vi "Main UI.vi"() -> ()   [LabVIEW 2021, in "Model.lvlib" / "Model.lvclass"]
uses:
  Model.lvclass
  <vilib>/OPCUA/controls/Subscription Data Change.ctl
  <vilib>/OPCUA/controls/NodeId.ctl
  <vilib>/OPCUA/controls/Data Type.ctl
  <vilib>/OPCUA/controls/OPC UA StatusCode.ctl
  Model.lvclass/Model.ctl
  <userlib>/John_Lib/Control/Panel State.ctl
  4ea6d537-f583-4af7-96b6-6e87ab69176a.vi
  dc795a0a-56a2-4742-a88d-ac9ee3460b1e.vi
  c0b4bdcd-4b65-4d6d-9257-8d5db7939309.vi
  005296f9-3097-4282-8b9c-b94103fb0c3d.vi
  921fea1b-c06a-452a-ac70-ed1835565b05.vi
  3e3e7c9d-885d-4de5-9ea6-85f2850c837d.vi
  cba7e740-a3a4-4717-84ae-86dbe1cc8337.vi
  <userlib>/John_Lib/OPCUA/UA Read Varient.vi
  adfd9d9b-45c5-4f5b-a64f-74c91a2677a3.vi
  <userlib>/John_Lib/AMC_FW/Send Local Message.vi
  <userlib>/John_Lib/AMC_FW/Read Next Message.vi
  <userlib>/John_Lib/AMC_FW/Parse State Queue__JKI.vi
  <userlib>/John_Lib/AMC_FW/Create Single Message.vi
  <userlib>/John_Lib/AMC_FW/Update Message Routing Info.vi
  <userlib>/John_Lib/AMC_FW/Read Termination Message.vi
  <vilib>/Utility/Data Type/Get Type Information.vi
  <userlib>/John_Lib/AMC_FW/String to Array.vi
  <userlib>/John_Lib/String/DBL to String.vi
  <userlib>/John_Lib/AMC_FW/Send Message.vi
  <userlib>/John_Lib/AMC_FW/Globals.vi
  <vilib>/Utility/error.llb/Trim Whitespace.vi
  <userlib>/John_Lib/OPCUA/add NameSpace for single NoteID.vi
  <vilib>/OPCUA/client/internal/Read.vi
  <vilib>/OPCUA/client/internal/Read Variant.vi
  <userlib>/John_Lib/OPCUA/OPCUA.lvclass
  <userlib>/John_Lib/AMC_FW/AMC_FW.lvlib
  <userlib>/John_Lib/TopPath/TopPath.lvlib
panel:
  in  "stop":bool
  out "data change":T1[](array[typedef]) {"data type" items=["Boolean"=1, "SByte"=2, "Byte"=3, "Int16"=4, "UInt16"=5, "Int32"=6, "UInt32"=7, "Int64"=8, "UInt64"=9, "Float"=10, "Double"=11, "String"=12, "DateTime"=13, "ByteString"=15, "Array of Boolean"=101, "Array of SByte"=102, "Array of Byte"=103, "Array of Int16"=104, "Array of UInt16"=105, "Array of Int32"=106, "Array of UInt32"=107, "Array of Int64"=108, "Array of UInt64"=109, "Array of Float"=110, "Array of Double"=111, "Array of String"=112, "Array of DateTime"=113, "Array of ByteString"=115, "Matrix of Boolean"=201, "Matrix of SByte"=202, "Matrix of Byte"=203, "Matrix of Int16"=204, "Matrix of UInt16"=205, "Matrix of Int32"=206, "Matrix of UInt32"=207, "Matrix of Int64"=208, "Matrix of UInt64"=209, "Matrix of Float"=210, "Matrix of Double"=211, "Matrix of String "=212, "Matrix of DateTime"=213, "Matrix of ByteString"=215]; "status code" items=["Good"=0, "Good_SubscriptionTransferred"=2949120, "Good_CompletesAsynchronously"=3014656, "Good_Overload"=3080192, "Good_Clamped"=3145728, "Good_LocalOverride"=9830400, "Good_EntryInserted"=10616832, "Good_EntryReplaced"=10682368, "Good_NoData"=10813440, "Good_MoreData"=10878976, "Good_CommunicationEvent"=10944512, "Good_ShutdownEvent"=11010048, "Good_CallAgain"=11075584, "Good_NonCriticalTimeout"=11141120, "Good_ResultsMayBeIncomplete"=12189696, "Good_DataIgnored"=14221312, "Uncertain"=1073741824, "Uncertain_ReferenceOutOfServer"=1080819712, "Uncertain_NoCommunicationLastUsableValue"=1083113472, "Uncertain_LastUsableValue"=1083179008, "Uncertain_SubstituteValue"=1083244544, "Uncertain_InitialValue"=1083310080, "Uncertain_SensorNotAccurate"=1083375616, "Uncertain_EngineeringUnitsExceeded"=1083441152, "Uncertain_SubNormal"=1083506688, "Uncertain_DataSubNormal"=1084489728, "Uncertain_ReferenceNotDeleted"=1086062592, "Uncertain_NotAllNodesAvailable"=1086324736, "Bad"=2147483648, "Bad_UnexpectedError"=2147549184, "Bad_InternalError"=2147614720, "Bad_OutOfMemory"=2147680256, "Bad_ResourceUnavailable"=2147745792, "Bad_CommunicationError"=2147811328, "Bad_EncodingError"=2147876864, "Bad_DecodingError"=2147942400, "Bad_EncodingLimitsExceeded"=2148007936, "Bad_UnknownResponse"=2148073472, "Bad_Timeout"=2148139008, "Bad_ServiceUnsupported"=2148204544, "Bad_Shutdown"=2148270080, "Bad_ServerNotConnected"=2148335616, "Bad_ServerHalted"=2148401152, "Bad_NothingToDo"=2148466688, "Bad_TooManyOperations"=2148532224, "Bad_DataTypeIdUnknown"=2148597760, "Bad_CertificateInvalid"=2148663296, "Bad_SecurityChecksFailed"=2148728832, "Bad_CertificateTimeInvalid"=2148794368, "Bad_CertificateIssuerTimeInvalid"=2148859904, "Bad_CertificateHostNameInvalid"=2148925440, "Bad_CertificateUriInvalid"=2148990976, "Bad_CertificateUseNotAllowed"=2149056512, "Bad_CertificateIssuerUseNotAllowed"=2149122048, "Bad_CertificateUntrusted"=2149187584, "Bad_CertificateRevocationUnknown"=2149253120, "Bad_CertificateIssuerRevocationUnknown"=2149318656, "Bad_CertificateRevoked"=2149384192, "Bad_CertificateIssuerRevoked"=2149449728, "Bad_UserAccessDenied"=2149515264, "Bad_IdentityTokenInvalid"=2149580800, "Bad_IdentityTokenRejected"=2149646336, "Bad_SecureChannelIdInvalid"=2149711872, "Bad_InvalidTimestamp"=2149777408, "Bad_NonceInvalid"=2149842944, "Bad_SessionIdInvalid"=2149908480, "Bad_SessionClosed"=2149974016, "Bad_SessionNotActivated"=2150039552, "Bad_SubscriptionIdInvalid"=2150105088, "Bad_RequestHeaderInvalid"=2150236160, "Bad_TimestampsToReturnInvalid"=2150301696, "Bad_RequestCancelledByClient"=2150367232, "Bad_NoCommunication"=2150694912, "Bad_WaitingForInitialData"=2150760448, "Bad_NodeIdInvalid"=2150825984, "Bad_NodeIdUnknown"=2150891520, "Bad_AttributeIdInvalid"=2150957056, "Bad_IndexRangeInvalid"=2151022592, "Bad_IndexRangeNoData"=2151088128, "Bad_DataEncodingInvalid"=2151153664, "Bad_DataEncodingUnsupported"=2151219200, "Bad_NotReadable"=2151284736, "Bad_NotWritable"=2151350272, "Bad_OutOfRange"=2151415808, "Bad_NotSupported"=2151481344, "Bad_NotFound"=2151546880, "Bad_ObjectDeleted"=2151612416, "Bad_NotImplemented"=2151677952, "Bad_MonitoringModeInvalid"=2151743488, "Bad_MonitoredItemIdInvalid"=2151809024, "Bad_MonitoredItemFilterInvalid"=2151874560, "Bad_MonitoredItemFilterUnsupported"=2151940096, "Bad_FilterNotAllowed"=2152005632, "Bad_StructureMissing"=2152071168, "Bad_EventFilterInvalid"=2152136704, "Bad_ContentFilterInvalid"=2152202240, "Bad_FilterOperandInvalid"=2152267776, "Bad_ContinuationPointInvalid"=2152333312, "Bad_NoContinuationPoints"=2152398848, "Bad_ReferenceTypeIdInvalid"=2152464384, "Bad_BrowseDirectionInvalid"=2152529920, "Bad_NodeNotInView"=2152595456, "Bad_ServerUriInvalid"=2152660992, "Bad_ServerNameMissing"=2152726528, "Bad_DiscoveryUrlMissing"=2152792064, "Bad_SempahoreFileMissing"=2152857600, "Bad_RequestTypeInvalid"=2152923136, "Bad_SecurityModeRejected"=2152988672, "Bad_SecurityPolicyRejected"=2153054208, "Bad_TooManySessions"=2153119744, "Bad_UserSignatureInvalid"=2153185280, "Bad_ApplicationSignatureInvalid"=2153250816, "Bad_NoValidCertificates"=2153316352, "Bad_RequestCancelledByRequest"=2153381888, "Bad_ParentNodeIdInvalid"=2153447424, "Bad_ReferenceNotAllowed"=2153512960, "Bad_NodeIdRejected"=2153578496, "Bad_NodeIdExists"=2153644032, "Bad_NodeClassInvalid"=2153709568, "Bad_BrowseNameInvalid"=2153775104, "Bad_BrowseNameDuplicated"=2153840640, "Bad_NodeAttributesInvalid"=2153906176, "Bad_TypeDefinitionInvalid"=2153971712, "Bad_SourceNodeIdInvalid"=2154037248, "Bad_TargetNodeIdInvalid"=2154102784, "Bad_DuplicateReferenceNotAllowed"=2154168320, "Bad_InvalidSelfReference"=2154233856, "Bad_ReferenceLocalOnly"=2154299392, "Bad_NoDeleteRights"=2154364928, "Bad_ServerIndexInvalid"=2154430464, "Bad_ViewIdUnknown"=2154496000, "Bad_TooManyMatches"=2154627072, "Bad_QueryTooComplex"=2154692608, "Bad_NoMatch"=2154758144, "Bad_MaxAgeInvalid"=2154823680, "Bad_HistoryOperationInvalid"=2154889216, "Bad_HistoryOperationUnsupported"=2154954752, "Bad_WriteNotSupported"=2155020288, "Bad_TypeMismatch"=2155085824, "Bad_MethodInvalid"=2155151360, "Bad_ArgumentsMissing"=2155216896, "Bad_TooManySubscriptions"=2155282432, "Bad_TooManyPublishRequests"=2155347968, "Bad_NoSubscription"=2155413504, "Bad_SequenceNumberUnknown"=2155479040, "Bad_MessageNotAvailable"=2155544576, "Bad_InsufficientClientProfile"=2155610112, "Bad_TcpServerTooBusy"=2155675648, "Bad_TcpMessageTypeInvalid"=2155741184, "Bad_TcpSecureChannelUnknown"=2155806720, "Bad_TcpMessageTooLarge"=2155872256, "Bad_TcpNotEnoughResources"=2155937792, "Bad_TcpInternalError"=2156003328, "Bad_TcpEndpointUrlInvalid"=2156068864, "Bad_RequestInterrupted"=2156134400, "Bad_RequestTimeout"=2156199936, "Bad_SecureChannelClosed"=2156265472, "Bad_SecureChannelTokenUnknown"=2156331008, "Bad_SequenceNumberInvalid"=2156396544, "Bad_ConfigurationError"=2156462080, "Bad_NotConnected"=2156527616, "Bad_DeviceFailure"=2156593152, "Bad_SensorFailure"=2156658688, "Bad_OutOfService"=2156724224, "Bad_DeadbandFilterInvalid"=2156789760, "Bad_RefreshInProgress"=2157379584, "Bad_ConditionAlreadyDisabled"=2157445120, "Bad_ConditionDisabled"=2157510656, "Bad_EventIdUnknown"=2157576192, "Bad_NoData"=2157641728, "Bad_DataLost"=2157772800, "Bad_DataUnavailable"=2157838336, "Bad_EntryExists"=2157903872, "Bad_NoEntryExists"=2157969408, "Bad_TimestampNotSupported"=2158034944, "Bad_InvalidArgument"=2158690304, "Bad_ConnectionRejected"=2158755840, "Bad_Disconnect"=2158821376, "Bad_ConnectionClosed"=2158886912, "Bad_InvalidState"=2158952448, "Bad_EndOfStream"=2159017984, "Bad_NoDataAvailable"=2159083520, "Bad_WaitingForResponse"=2159149056, "Bad_OperationAbandoned"=2159214592, "Bad_ExpectedStreamToBlock"=2159280128, "Bad_WouldBlock"=2159345664, "Bad_SyntaxError"=2159411200, "Bad_MaxConnectionsReached"=2159476736, "Bad_RequestTooLarge"=2159542272, "Bad_ResponseTooLarge"=2159607808, "Bad_EventNotAcknowledgeable"=2159738880, "Bad_InvalidTimestampArgument"=2159869952, "Bad_ProtocolVersionUnsupported"=2159935488, "Bad_StateNotActive"=2160001024, "Bad_FilterOperatorInvalid"=2160132096, "Bad_FilterOperatorUnsupported"=2160197632, "Bad_FilterOperandCountMismatch"=2160263168, "Bad_FilterElementInvalid"=2160328704, "Bad_FilterLiteralInvalid"=2160394240, "Bad_IdentityChangeNotSupported"=2160459776, "Bad_NotTypeDefinition"=2160590848, "Bad_ViewTimestampInvalid"=2160656384, "Bad_ViewParameterMismatch"=2160721920, "Bad_ViewVersionInvalid"=2160787456, "Bad_ConditionAlreadyEnabled"=2160852992, "Bad_DialogNotActive"=2160918528, "Bad_DialogResponseInvalid"=2160984064, "Bad_ConditionBranchAlreadyAcked"=2161049600, "Bad_ConditionBranchAlreadyConfirmed"=2161115136, "Bad_ConditionAlreadyShelved"=2161180672, "Bad_ConditionNotShelved"=2161246208, "Bad_ShelvingTimeOutOfRange"=2161311744, "Bad_AggregateListMismatch"=2161377280, "Bad_AggregateNotSupported"=2161442816, "Bad_AggregateInvalidInputs"=2161508352, "Bad_BoundNotFound"=2161573888, "Bad_BoundNotSupported"=2161639424, "Bad_AggregateConfigurationRejected"=2161770496, "Bad_TooManyMonitoredItems"=2161836032]}
  out "value":variant
  in  "node ID":string
  in  "error out":errorcluster
  out "Error Out":errorcluster
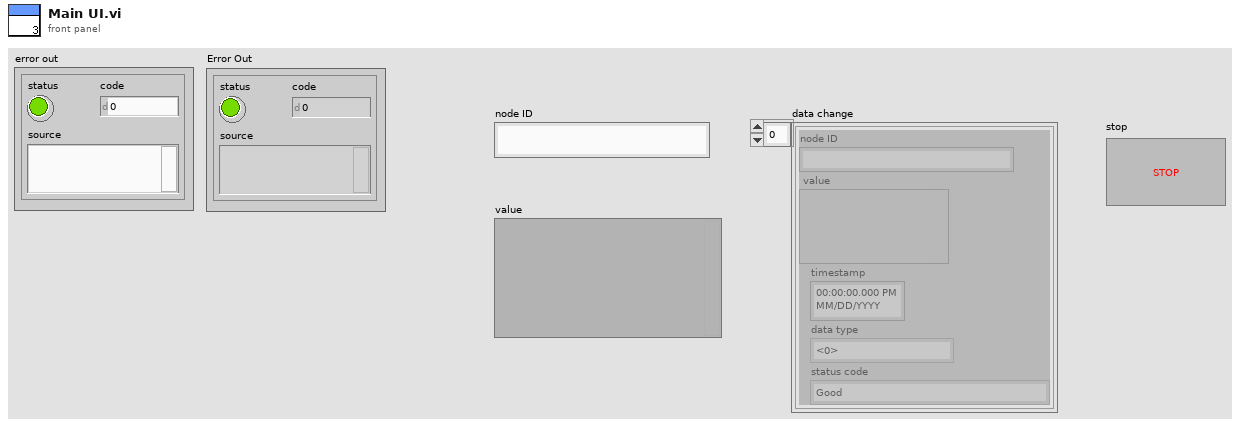
[diagram p1: front panel]
types:
  T1 = typedef "Subscription Data Change.ctl" = cluster{"node ID":T2, " value":variant, "timestamp":timestamp, "data type":T3, "status code":T4}
  T2 = typedef "NodeId.ctl" = string
  T3 = typedef "Data Type.ctl" = u16
  T4 = typedef "OPC UA StatusCode.ctl" = u32
  T5 = typedef "OPCUA.lvlib/OPCUA.lvclass/OPCUA Even.ctl" = cluster{"OPC UA data change":refnum<user-event>, "ReSubscribtion":refnum<user-event>}
  T6 = typedef "Model.lvlib/Model.lvclass/Evens.ctl" = cluster{"NotifyIcon":refnum<user-event>, "Stop":refnum<user-event>}
  T7 = typedef "AMC_FW.lvlib/Queue.ctl" = cluster{"Q":T8, "Name":string}
  T8 = typedef "AMC_FW.lvlib/Message Queue.ctl" = refnum<queue>
  T9 = enum32{"invalid app kind", "Development System", "Run Time System", "Student Edition", "Embedded LabVIEW", "Evaluation", "Custom"}
  T10 = typedef "Panel State.ctl" = string
  T11 = typedef "Model.lvlib/Model.lvclass/DVR.ctl" = cluster{"JKI_Network_Streams":refnum<class "NetworkConnection.lvclass">, "AMC Q":T12}
  T12 = typedef "Model.lvlib/Model.lvclass/AMC Q.ctl" = cluster{"Main":T7, "OPCUA":T7, "NetworkSteam":T7}
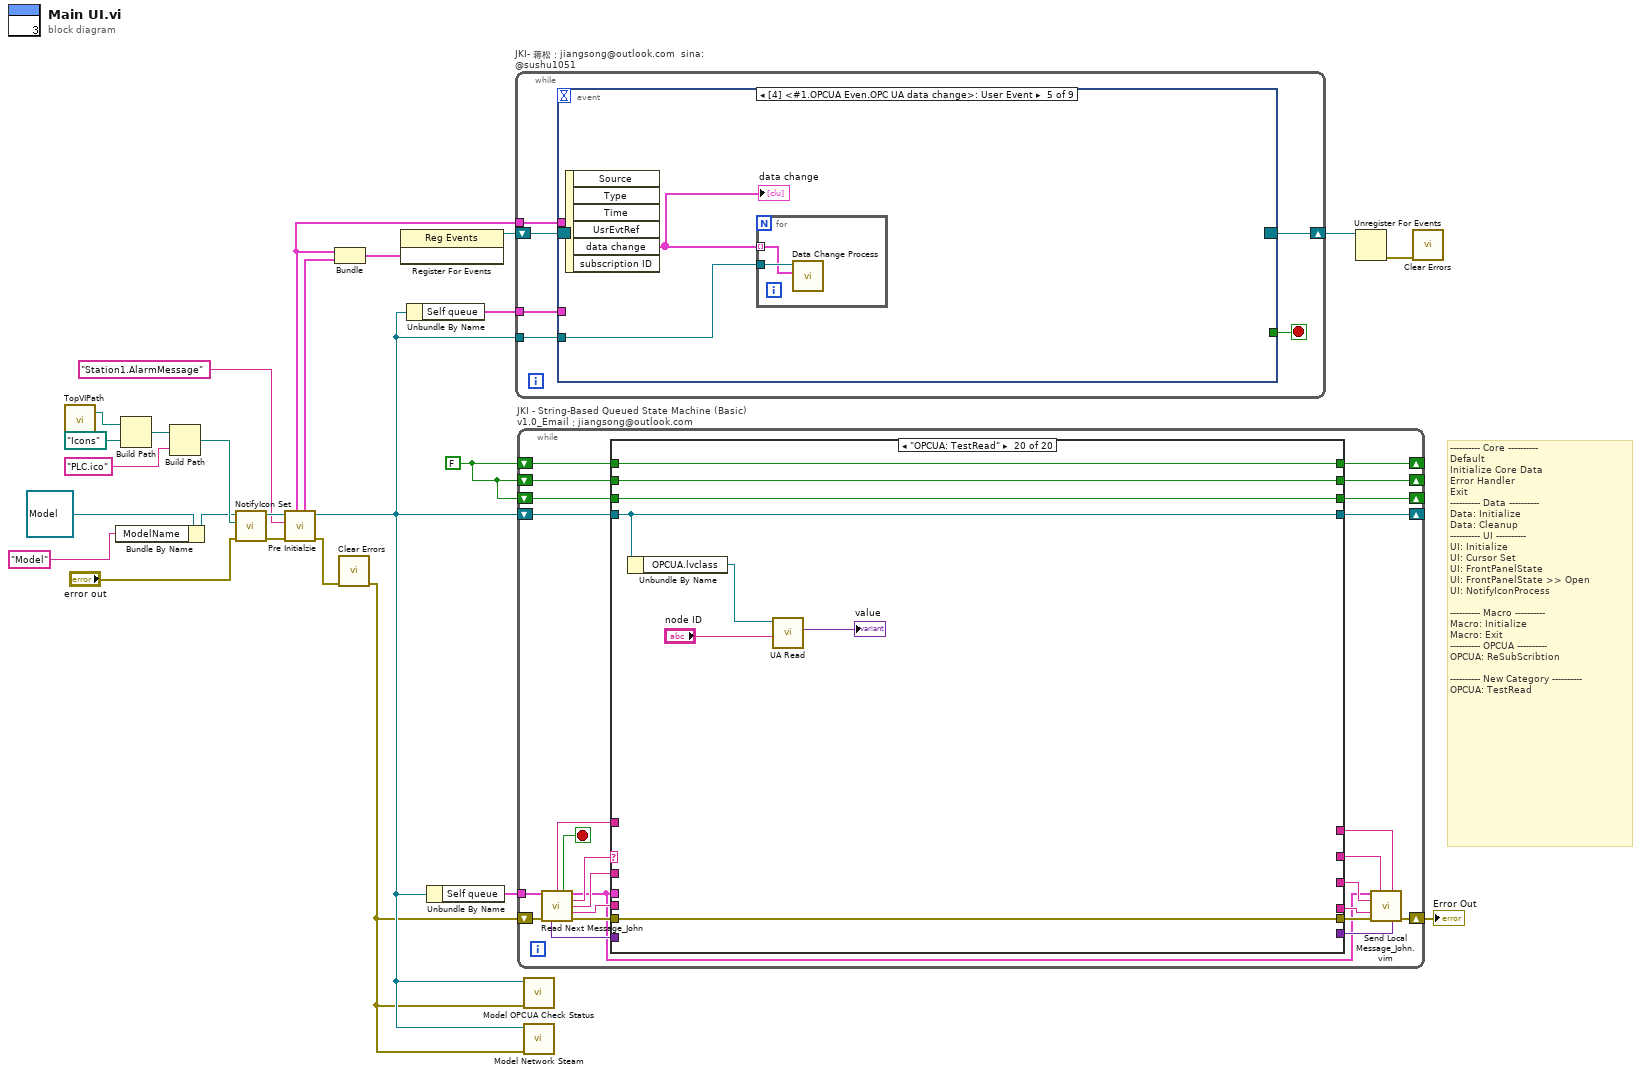
[diagram p0: block diagram]
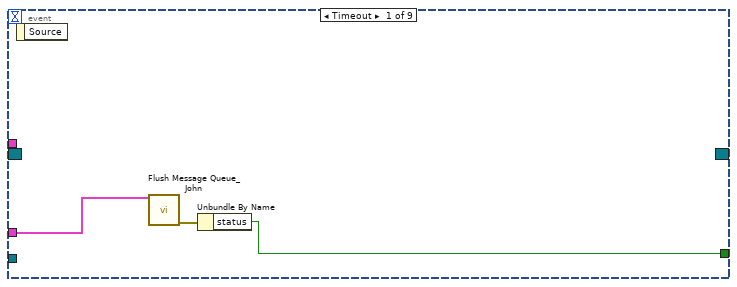
[diagram p2: hidden frame]
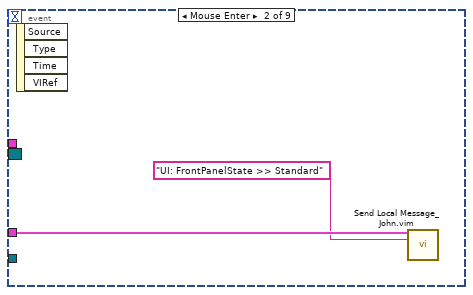
[diagram p3: hidden frame]
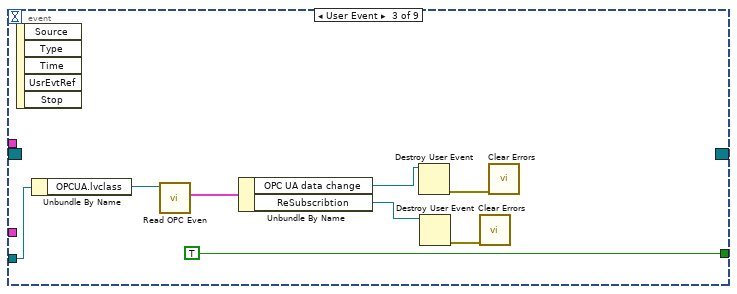
[diagram p4: hidden frame]
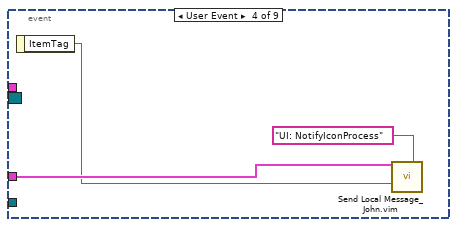
[diagram p5: hidden frame]
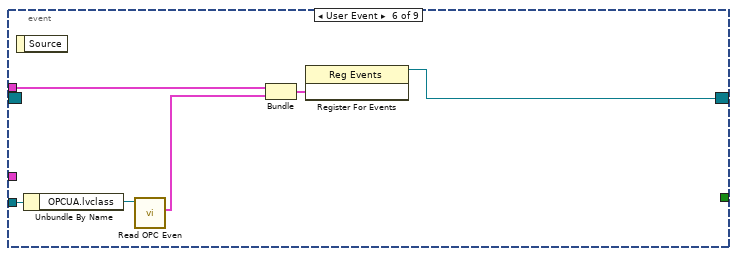
[diagram p6: hidden frame]
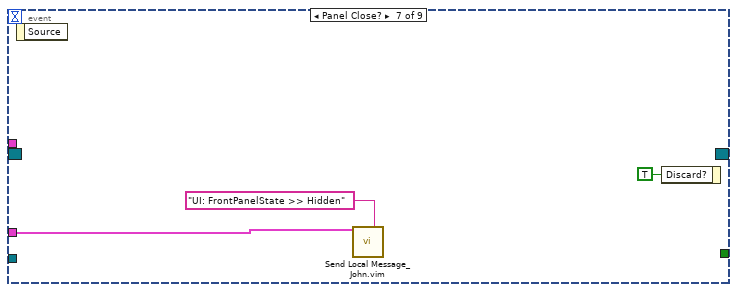
[diagram p7: hidden frame]
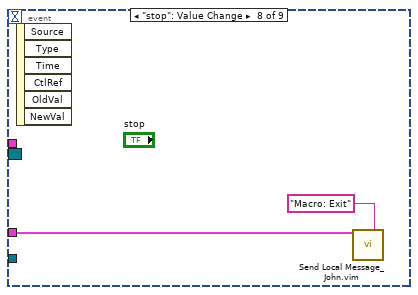
[diagram p8: hidden frame]
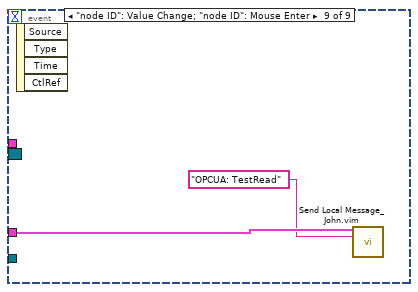
[diagram p9: hidden frame]
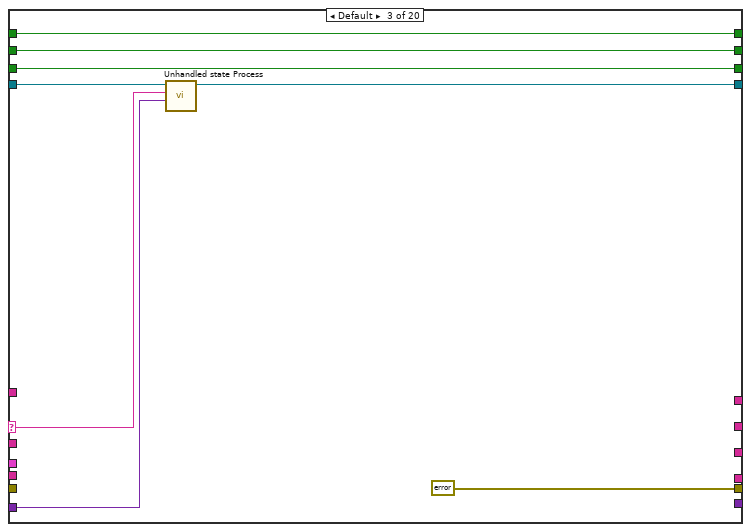
[diagram p12: hidden frame]
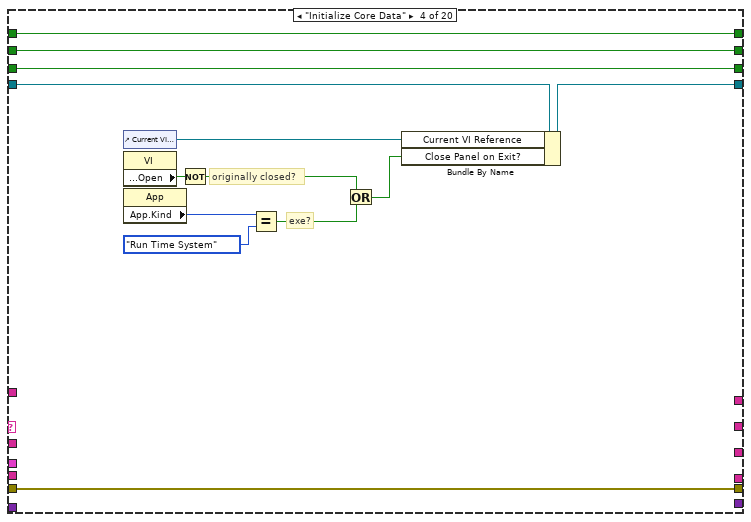
[diagram p13: hidden frame]
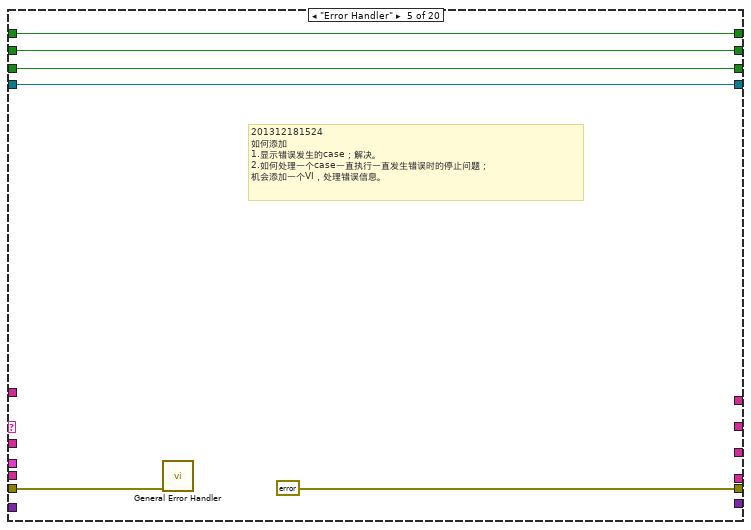
[diagram p14: hidden frame]
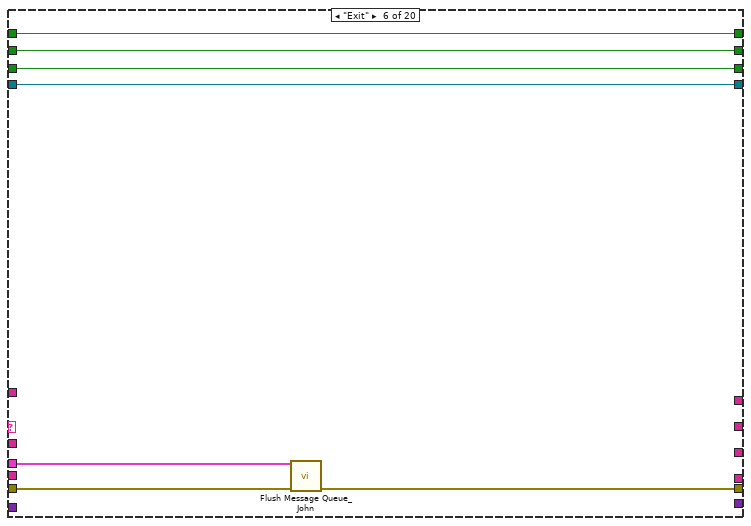
[diagram p15: hidden frame]
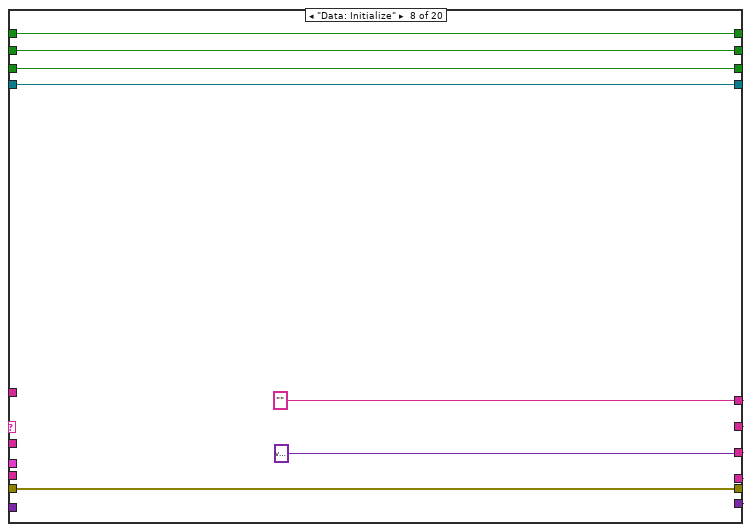
[diagram p17: hidden frame]
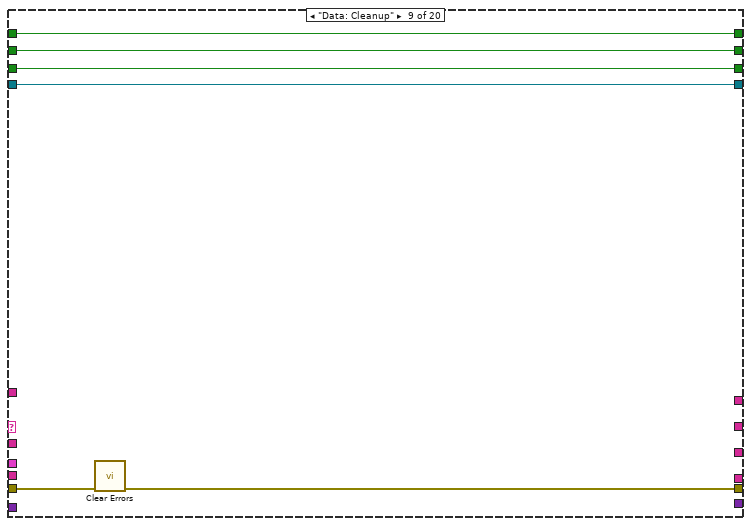
[diagram p18: hidden frame]
diagram:
  w17 = FALSE
  # "---------- Core ----------\nDefault\nInitialize Core Data\nError Handler\nExit\n---------- Data ----------\nData: Initialize\nData: Cleanup\n---------- UI ----------\nUI: Initialize\nUI: Cursor Set\nUI: FrontPanelState\nUI: FrontPanelState >> Open\nUI: NotifyIconProcess\n\n---------- Macro ----------\nMacro: Initialize\nMacro: Exit\n---------- OPCUA ----------\nOPCUA: ReSubScribtion\n\n---------- New Category ----------\nOPCUA: TestRead"
  n1 = call <userlib>:"TopVIPath.vi"() -> ("ConfigFile path"=w14:path)  [unwired: 1 in, 2 out]
  n2 = Bundle By Name(cluster=refnum<class "Model.lvclass"> refnum ("Model.lvlib:Model.lvclass"), "ModelName"="Model" ("Icon Name")) -> (w2:refnum<class "Model.lvclass">)
  n3 = Build Path(base path=w14, name or relative path=path "Icons") -> (appended path=w13:path)
  n4 = Build Path(base path=w13, name or relative path="PLC.ico") -> (appended path=w18:path)
  n5 = call "NotifyIcon Set.vi"("error in (no error)"="error out", "Icon path"=w18, "Model in"=w2) -> ("error out"=w15:errorcluster, "Model out"=w16:refnum<class "Model.lvclass">)  [unwired: 7 in]
  n6 = call "Pre Initialzie.vi"("error in (no error)"=w15, "SUbscription Node IDs"="Station1.AlarmMessage", "Model in"=w16) -> ("error out"=w5:errorcluster, "Model out"=w4:refnum<class "Model.lvclass">, "OPCUA Even"=w11:T5, "Evens"=w8:T6)  [unwired: 5 in]
  n7 = Bundle("Evens"=w8, "OPCUA Even"=w11) -> (w12:cluster{"Evens":T6, "OPCUA Even":T5})  [unwired: 1 in]
  n8 = call <vilib>:"Clear Errors.vi"("error in (no error)"=w5) -> ("error out"=w3:errorcluster)  [unwired: 5 in, 1 out]
  n9 = register-events(w12) -> (reference out=w23:refnum<event-registration>)  [unwired: 2 in, 1 out]
  n10 = Unbundle By Name(w4) -> ("Self queue"=w6:T7)
  n11 = Unbundle By Name(w4) -> ("Self queue"=w7:T7)
  n12 = while "JKI- 蒋松：jiangsong@outlook.com  sina: @sushu1051" {
    tunnel: w6 -> [w31]
    shift-right: [w28] -> w24
    shift-left: w23 -> [w29]
    tunnel: w4 -> [w27]
    tunnel: w8 -> [w26]
    stop <- w30 stop-if-true
    n13 = event shown="[4] <#1.OPCUA Even.OPC UA data change>: User Event" {
      selector: w29 -> [_ _ _ _ _ _ _ _ _]
      dyn-events: [_ _ _ _ _ w55 _ _ _] -> w28
      timeout: _ -> [_ _ _ _ _ _ _ _ _]
      tunnel: w31 -> [w33 w37 _ w48 _ _ w60 w63 w65]
      tunnel: [w32 _ TRUE ("status") _ _ _ _ _ _] -> w30
      tunnel: w27 -> [_ _ w43 _ w49 w58 _ _ _]
      tunnel: w26 -> [_ _ _ _ _ w56 _ _ _]
      event Timeout {
        n14 = event-data() -> ()  [unwired: 1 in, 1 out]
        n15 = call <userlib>:"Flush Message Queue_John.vi"("Queue In"=w33) -> ("error out"=w35:errorcluster)  [unwired: 12 in, 2 out]
        n16 = Unbundle By Name(w35) -> ("status"=w32:bool)
        n17 = Format Date/Time String(time format string (%c)="%Y-%m-%d\n%H : %M : %S") -> ()  [unwired: 2 in, 1 out]
      }
      event Mouse Enter {
        n18 = event-data() -> ()  [unwired: 1 in, 4 out]
        n19 = call "Send Local Message_John.vim"("Queue In"=w37, "Elements at Back"="UI: FrontPanelState >> Standard") -> ()  [unwired: 11 in, 3 out]
      }
      event User Event {
        n20 = event-data() -> ()  [unwired: 1 in, 5 out]
        n21 = Unbundle By Name(w43) -> ("OPCUA.lvclass"=w44:refnum<class "OPCUA.lvclass">)
        n22 = call <userlib>:"Read OPC Even.vi"("OPCUA in"=w44) -> ("Even"=w39:T5)  [unwired: 8 in, 2 out]
        n23 = Unbundle By Name(w39) -> ("OPC UA data change"=w42:refnum<user-event>, "ReSubscribtion"=w41:refnum<user-event>)
        n24 = Destroy User Event(user event=w42) -> (error out=w40:errorcluster)  [unwired: 1 in]
        n25 = Destroy User Event(user event=w41) -> (error out=w38:errorcluster)  [unwired: 1 in]
        n26 = call <vilib>:"Clear Errors.vi"("error in (no error)"=w38) -> ()  [unwired: 5 in, 2 out]
        n27 = call <vilib>:"Clear Errors.vi"("error in (no error)"=w40) -> ()  [unwired: 5 in, 2 out]
      }
      event User Event {
        n28 = event-data() -> ("ItemTag"=w46:string)  [unwired: 1 in]
        n29 = call "Send Local Message_John.vim"("Queue In"=w48, "Elements in Front"="UI: NotifyIconProcess", "message value"=w46) -> ()  [unwired: 10 in, 3 out]
      }
      event User Event {
        n30 = event-data() -> ("data change"=w50:T1[])  [unwired: 1 in, 5 out]
        "data change" <- w50
        n31 = for {
          tunnel: w50 -> [w51] mode=indexing
          tunnel: w49 -> [w52]
          n32 = call "Data Change Process.vi"("data change"=w51, "Model in"=w52) -> ()  [unwired: 8 in, 2 out]
        }
      }
      event User Event {
        n33 = event-data() -> ()  [unwired: 1 in, 1 out]
        n34 = Unbundle By Name(w58) -> ("OPCUA.lvclass"=w54:refnum<class "OPCUA.lvclass">)
        n35 = call <userlib>:"Read OPC Even.vi"("OPCUA in"=w54) -> ("Even"=w53:T5)  [unwired: 8 in, 2 out]
        n36 = Bundle("Evens"=w56, "Even"=w53) -> (w57:cluster{"Evens":T6, "Even":T5})  [unwired: 1 in]
        n37 = register-events(w57) -> (reference out=w55:refnum<event-registration>)  [unwired: 2 in, 1 out]
      }
      event Panel Close? {
        n38 = event-data() -> ()  [unwired: 1 in, 1 out]
        n39 = call "Send Local Message_John.vim"("Queue In"=w60, "Elements in Front"="UI: FrontPanelState >> Hidden") -> ()  [unwired: 11 in, 3 out]
        n40 = event-data("Discard?"=TRUE) -> ()  [unwired: 1 in, 1 out]
      }
      event "stop": Value Change {
        n41 = event-data() -> ()  [unwired: 1 in, 6 out]
        n42 = call "Send Local Message_John.vim"("Queue In"=w63, "Elements in Front"="Macro: Exit") -> ()  [unwired: 11 in, 3 out]
      }
      event "node ID": Value Change; "node ID": Mouse Enter {
        n43 = event-data() -> ()  [unwired: 1 in, 4 out]
        n44 = call "Send Local Message_John.vim"("Queue In"=w65, "Elements at Back"="OPCUA: TestRead" ("Elements in Front")) -> ()  [unwired: 11 in, 3 out]
      }
    }
  }
  n45 = while "JKI - String-Based Queued State Machine (Basic) v1.0_Email：jiangsong@outlook.com" {
    shift-right: [w75] -> w22
    shift-left: w3 -> [w84]
    shift-right: [w89] -> _
    shift-left: w17 -> [w90]
    shift-right: [w85] -> _
    shift-left: w4 -> [w78]
    shift-right: [w86] -> _
    shift-left: w17 -> [w76]
    shift-right: [w87] -> _
    shift-left: w17 -> [w88]
    tunnel: w7 -> [w81]
    stop <- w67 stop-if-true
    n46 = call <userlib>:"Read Next Message_John.vi"("Queue In"=w81, "error in"=w84) -> ("Previous State + Arguments"=w77:string, "exit process?"=w67:bool, "Queue Out"=w66:T7, "Current State"=w82:string, "Arguments"=w80:string, "message value"=w79:string, "variant"=w68:variant, "error out"=w83:errorcluster)  [unwired: 4 in, 2 out]
    n47 = case shown="\"OPCUA: TestRead\"" w82 {
      selector: w82 -> [_ _ w102 _ _ _ _ _ _ _ _ _ _ _ _ _ w213 _ _ _]
      tunnel: w66 -> [_ _ _ _ _ w129 _ _ _ _ _ _ _ _ _ w196 w224 _ _ _]
      tunnel: w79 -> [_ _ _ _ _ _ _ _ _ _ _ _ _ w185 _ _ _ _ _ _]
      tunnel: [w91 w100 errorcluster {"status"=FALSE, "code"=0, "source"=""} ("error out") w119 errorcluster {"status"=FALSE, "code"=0, "source"=""} ("error out") w130 w136 w144 w149 w154 w160 w165 w177 w184 w192 w202 w222 w248 w258 w266] -> w74
      tunnel: w83 -> [w91 w100 _ w119 w123 w131 w136 w144 w147 w154 w160 w166 w178 _ w192 w202 w223 w248 w258 w266]
      tunnel: w90 -> [w95 w99 w108 w121 w127 w134 w139 w146 w150 w157 w162 w169 w183 w190 w195 w205 w235 w250 w257 w265]
      tunnel: [w95 w99 w108 w121 w127 w134 w139 w146 w150 w157 w162 w169 w183 w190 w195 w205 w235 w250 w257 w265] -> w89
      tunnel: w88 -> [w94 w98 w107 w120 w124 w133 w138 w145 w152 w156 w158 w168 w182 w189 w194 w204 w233 w249 w256 w264]
      tunnel: w76 -> [w93 w96 w105 w118 w125 w132 w135 w143 w148 w153 w159 w164 w181 w188 w191 w203 w234 w246 w255 w263]
      tunnel: w78 -> [w92 w97 w103 w110 w126 w128 w137 w141 w151 w155 w161 w167 w180 w186 w193 w197 w216 w247 w253 w262]
      tunnel: [w94 w98 w107 w120 w124 w133 w138 w145 w152 w156 w158 w168 w182 w189 w194 w204 w233 w249 w256 w264] -> w87
      tunnel: [w93 w96 w105 w118 w125 w132 w135 w143 w148 w153 w159 w164 w181 w188 w191 w203 w234 w246 w255 w263] -> w86
      tunnel: [w92 w97 w104 w109 w126 w128 w137 w141 w151 w155 w161 w167 w180 w187 w193 w200 w217 w247 w254 w262] -> w85
      tunnel: w80 -> [_ _ _ _ _ _ _ _ _ _ _ w163 w174 _ _ _ _ _ _ _]
      tunnel: w77 -> [_ _ _ _ _ _ _ _ _ _ _ _ _ _ _ _ _ _ _ _]
      tunnel: [_ _ _ _ _ _ _ w142 _ _ _ _ _ _ _ _ _ _ _ _] -> w73
      tunnel: [_ _ _ _ _ _ _ w142 _ _ _ _ _ _ _ _ w225 _ _ _] -> w72
      tunnel: [_ _ _ _ _ _ _ w142 _ _ _ _ _ _ _ "Data: Initialize\nInitialize Core Data\nUI: Initialize\n" _ _ _ _] -> w71
      tunnel: [_ _ _ _ _ _ _ w142 _ _ _ _ _ _ _ _ _ _ _ _] -> w70
      tunnel: [_ _ _ _ _ _ _ variant ("variant") _ _ _ _ _ _ _ _ _ _ _ _] -> w69
      tunnel: w68 -> [_ _ w101 _ _ _ _ _ _ _ _ _ _ _ _ _ _ _ _ _]
      frame "", "Idle" {
      }
      frame "---------- Core ----------" {
      }
      frame Default {
        n48 = call "Unhandled state Process.vi"("variant"=w101, "Unhandled state Case Name"=w102, "Model in"=w103) -> ("Model out"=w104:refnum<class "Model.lvclass">)  [unwired: 7 in, 1 out]
      }
      frame "Initialize Core Data" {
        # "originally closed?"
        # "exe?"
        n49 = control-ref of="Current VI Reference"() -> (w117:refnum<vi>)
        n50 = property class="VI"() -> ("Front Panel.Open"=w111:bool)  [unwired: 2 in, 2 out]
        n51 = property class="App"() -> ("App.Kind"=w112:T9)  [unwired: 2 in, 2 out]
        n52 = Not(x=w111) -> (.not. x?=w114:bool)
        n53 = Equal?(x=w112, y=T9."Run Time System" ("Application:Kind")) -> (x = y?=w115:bool)
        n54 = Or(x=w114, y=w115) -> (x .or. y?=w116:bool)
        n55 = Bundle By Name(cluster=w110, "Current VI Reference"=w117, "Close Panel on Exit?"=w116) -> (w109:refnum<class "Model.lvclass">)
      }
      frame "Error Handler" {
        # "201312181524\n如何添加\n1.显示错误发生的case；解决。\n2.如何处理一个case一直执行一直发生错误时的停止问题；\n机会添加一个VI，处理错误信息。"
        n56 = call <vilib>:"General Error Handler.vi"("error in (no error)"=w123) -> ()  [unwired: 10 in, 5 out]
      }
      frame "Exit" {
        n57 = call <userlib>:"Flush Message Queue_John.vi"("Queue In"=w129, "error in"=w131) -> ("error out"=w130:errorcluster)  [unwired: 11 in, 2 out]
      }
      frame "---------- Data ----------" {
      }
      frame "Data: Initialize" {
        w142 = "" ("Elements in Front")
      }
      frame "Data: Cleanup" {
        n58 = call <vilib>:"Clear Errors.vi"("error in (no error)"=w147) -> ("error out"=w149:errorcluster)  [unwired: 5 in, 1 out]
      }
      frame "---------- UI ----------" {
      }
      frame "UI: Initialize" {
      }
      frame "UI: CursorSet" {
        # "Argument"
        n59 = case shown="\"Idle\", Default" w163 {
          tunnel: w166 -> [w171 w173]
          tunnel: [w170 w172] -> w165
          frame "Idle", Default {
            n60 = call <vilib>:"Unset Busy.vi"("error in (no error)"=w171) -> ("error out"=w170:errorcluster)  [unwired: 10 in]
          }
          frame "Busy" {
            n61 = call <vilib>:"Set Busy.vi"("error in (no error)"=w173) -> ("error out"=w172:errorcluster)  [unwired: 9 in, 1 out]
          }
        }
      }
      frame "UI: FrontPanelState" {
        # "Argument"
        n62 = Unbundle By Name(w180) -> ("Current VI Reference"=w179:refnum<vi>)
        n63 = Type Cast(type=T10 "Standard" ("Argument"), x=w174) -> (*(type *) &x=w175:T10)
        n64 = call <userlib>:"Control Front Panel State.vi"("error out"=w178, "Argument"=w175, "Core.Current VI Reference"=w179) -> ("error out"=w177:errorcluster)  [unwired: 7 in, 1 out]
      }
      frame "UI: NotifyIconProcess" {
        n65 = call "NotifyIcon Process.vi"("ItemTag"=w185, "Model in"=w186) -> ("error out"=w184:errorcluster, "Model out"=w187:refnum<class "Model.lvclass">)  [unwired: 8 in]
      }
      frame "---------- Macro ----------" {
      }
      frame "Macro: Initialize" {
        # "空白处添加各种状态"
        n66 = control-ref of="This VI"() -> (w199:refnum<vi>)
        n67 = Unbundle By Name(w197) -> ("DVR_Self"=w198:refnum<data-value>)
        n68 = in-place {
          in-place-border: w196 -> [w206]
          n69 = in-place-dvr #1(w198) -> (w208:T11)  [unwired: 1 out]
          n70 = Bundle By Name(cluster=w208, "AMC Q.Main"=w206) -> (w207:T11)
          n71 = in-place-dvr #1(w207) -> ()  [unwired: 2 out]
        }
        n72 = Bundle By Name(cluster=w197, "ActorVI Ref"=w199, "Self queue"=w196) -> (w200:refnum<class "Model.lvclass">)
      }
      frame "Macro: Exit" {
        n73 = Unbundle By Name(w216) -> ("Close Panel on Exit?"=w232:bool, "DVR_Self"=w212:refnum<data-value>)
        n74 = Unbundle By Name(w216) -> ("Stop"=w220:refnum<user-event>)
        n75 = call <userlib>:"Flush Message Queue_John.vi"("Queue In"=w224, "error in"=w223) -> ("error out"=w222:errorcluster)  [unwired: 11 in, 2 out]
        n76 = in-place {
          in-place-border: [w236] -> w211
          n77 = in-place-dvr #2(w212) -> (w236:T11)  [unwired: 1 out]
          n78 = in-place-dvr #2(w236) -> ()  [unwired: 2 out]
        }
        n79 = Generate User Event(user event=w220, event data cluster=FALSE ("event data")) -> (error out=w219:errorcluster)  [unwired: 2 in, 1 out]
        n80 = call "Stop Cores.vi"("error in (no error)"=w219, "Model in"=w216) -> ("Model out"=w217:refnum<class "Model.lvclass">)  [unwired: 8 in, 1 out]
        n81 = Unbundle By Name(w211) -> ("AMC Q.OPCUA"=w209:T7, "AMC Q.NetworkSteam"=w210:T7)
        n82 = call "Send Local Message_John.vim"("Queue In"=w209, "Elements in Front"=w213) -> ("error out"=w221:errorcluster)  [unwired: 11 in, 2 out]
        n83 = call <vilib>:"Clear Errors.vi"("error in (no error)"=w221) -> ("error out"=w215:errorcluster)  [unwired: 5 in, 1 out]
        n84 = Select(t="UI: FrontPanelState >> Close", s=w232, f="") -> (s? t:f=w231:string)
        n85 = call "Send Local Message_John.vim"("Queue In"=w210, "Elements in Front"=w213, "error in"=w215) -> ("error out"=w214:errorcluster)  [unwired: 10 in, 2 out]
        n86 = call <vilib>:"Clear Errors.vi"("error in (no error)"=w214) -> ()  [unwired: 5 in, 2 out]
        n87 = case shown="False" w232 {
          tunnel: w231 -> [w240 _]
          tunnel: "" -> [w241 w245]
          tunnel: "\r" -> [w239 w244]
          tunnel: "Data: Cleanup\nExit" -> [w238 w243]
          tunnel: [w237 w242] -> w225
          frame True {
            n88 = Concatenate Strings(w241, w239, w240, w239, w238) -> (w237:string)
          }
          frame False {
            n89 = Concatenate Strings(w245, w244, w243) -> (w242:string)
          }
        }
      }
      frame "---------- Control ----------" {
      }
      frame "OPCUA: ReSubScribtion" {
        n90 = Unbundle By Name(w253) -> ("OPCUA.lvclass"=w251:refnum<class "OPCUA.lvclass">)
        n91 = call <userlib>:"ReCreate Subscription.vi"("OPCUA in"=w251) -> ("OPCUA out"=w252:refnum<class "OPCUA.lvclass">)  [unwired: 7 in, 3 out]
        n92 = Bundle By Name(cluster=w253, "OPCUA.lvclass"=w252) -> (w254:refnum<class "Model.lvclass">)
      }
      frame "OPCUA: TestRead" {
        n93 = Unbundle By Name(w262) -> ("OPCUA.lvclass"=w261:refnum<class "OPCUA.lvclass">)
        n94 = call-poly <userlib>:"UA Read.vi"("node ID"="node ID", "OPCUA in"=w261) -> ("value"=→"value":variant)  [unwired: 5 in, 4 out]
      }
    }
    n95 = call "Send Local Message_John.vim"("Queue In"=w66, "receiver process (\"\" - local)"=w73, "Elements in Front"=w72, "Elements at Back"=w71, "message value"=w70, "error in"=w74, "variant"=w69) -> ("error out"=w75:errorcluster)  [unwired: 6 in, 2 out]
  }
  "Error Out" <- w22
  n96 = call "Model OPCUA Check Status.vi"("error in (no error)"=w3, "Model in"=w4) -> ()  [unwired: 9 in, 1 out]
  n97 = call "Model Network Steam.vi"("error in (no error)"=w3, "Model in"=w4) -> ()  [unwired: 9 in, 1 out]
  n98 = Unregister For Events(event registration refnum=w24) -> (error out=w25:errorcluster)  [unwired: 1 in]
  n99 = call <vilib>:"Clear Errors.vi"("error in (no error)"=w25) -> ()  [unwired: 5 in, 2 out]
